vi "simple_acquisition.vi"() -> ()   [LabVIEW 2015]
uses:
  <vilib>/userdefined/High Color/IMAQdx.ctl
  <vilib>/vision/driver/NI_Vision_Acquisition_Software.lvlib
  <resource>/objmgr/imaqdx.rc
panel:
  in  "ExposureTimeRawValue":dbl(slide)=2237.4518320560815 scale=1.0..100000.0
  in  "File Path Control":path
  in  "Camera":T1="cam4"
  out "Image source":T2(plugin-control)
  in  "Acquire Image":bool
  in  "Image Name":string
  in  "Image Format":string(combo)=".png"
  in  "Stop Button":bool
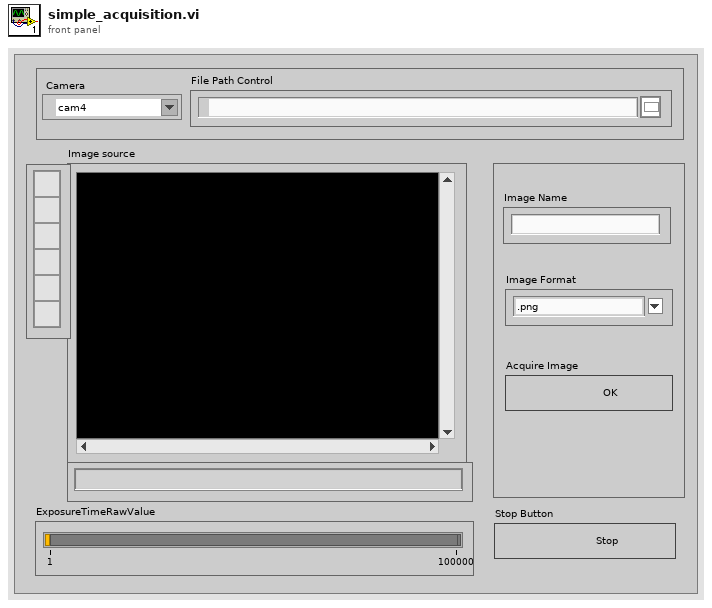
[diagram p1: front panel]
types:
  T1 = typedef "IMAQdx.ctl" = refnum<k21>
  T2 = typedef "IMAQ Image.ctl" = refnum<image>
  T3 = typedef "Image Type" = u32
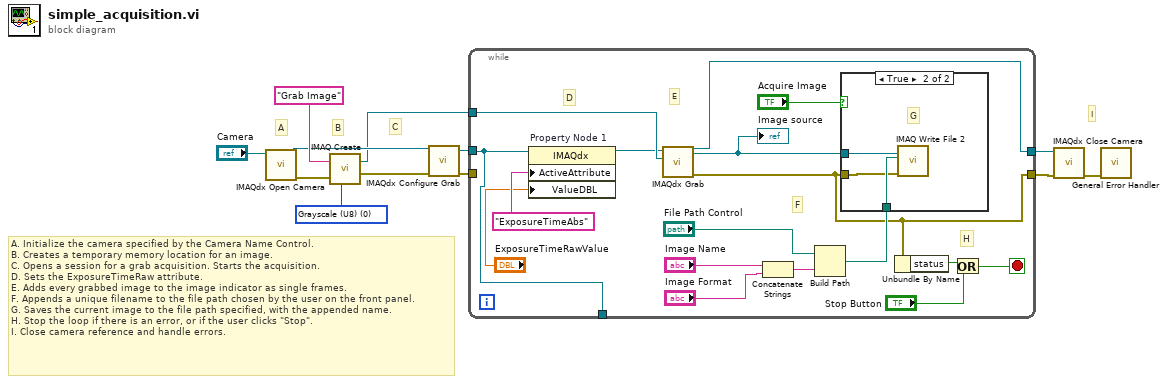
[diagram p0: block diagram]
diagram:
  w11 = T3 0 items=["Grayscale (U8)", "Grayscale (I16)", "Grayscale (SGL)", "Complex (CSG)", "RGB (U32)", "HSL (U32)", "RGB (U64)"] ("Image Type")
  # "I"
  # "C"
  # "A. Initialize the camera specified by the Camera Name Control.\nB. Creates a temporary memory location for an image.\nC. Opens a session for a grab acquisition. Starts the acquisition.\nD. Sets the ExposureTimeRaw attribute. \nE. Adds every grabbed image to the image indicator as single frames.\nF. Appends a unique filename to the file path chosen by the user on the front panel.\nG. Saves the current image to the file path specified, with the appended name.\nH. Stop the loop if there is an error, or if the user clicks \"Stop\".\nI. Close camera reference and handle errors."
  # "B"
  # "A"
  n1 = call <vilib>:"IMAQdx Open Camera.vi"("Session In"="Camera") -> ("error out"=w3:errorcluster, "Session Out"=w8:T1)  [unwired: 2 in, 7 out]
  n2 = call "IMAQ Create"("Image Name"="Grab Image", "Image Type"=w11, "error in (no error)"=w3) -> ("New Image"=w1:T2, "error out"=w10:errorcluster)  [unwired: 1 in, 1 out]
  n3 = call <vilib>:"IMAQdx Configure Grab.vi"("error in"=w10, "Session In"=w8) -> ("error out"=w2:errorcluster, "Session Out"=w4:T1)  [unwired: 8 out]
  n4 = while {
    tunnel: w2 -> [_]
    tunnel: w4 -> [w13]
    tunnel: [w19] -> w6
    tunnel: [w21] -> w5
    tunnel: w1 -> [w18]
    tunnel: [w13] -> _
    stop <- w23 stop-if-true
    # "H"
    # "F"
    # "E"
    # "D"
    n5 = property on="Property Node 1" class="IMAQdx"(reference=w13, "ActiveAttribute"="ExposureTimeAbs" ("String"), "ValueDBL"="ExposureTimeRawValue") -> (reference out=w17:T1)  [unwired: 1 in, 1 out]
    n6 = call <vilib>:"IMAQdx Grab.vi"("Image In"=w18, "Session In"=w17) -> ("error out"=w19:errorcluster, "Image Out"=w14:T2, "Session Out"=w21:T1)  [unwired: 2 in, 5 out]
    "Image source" <- w14
    n7 = Concatenate Strings("Image Name", "Image Format") -> (w29:string)
    n8 = Build Path(base path="File Path Control", name or relative path=w29) -> (appended path=w25:path)
    n9 = case shown="True" "Acquire Image" {
      tunnel: w14 -> [_ w30]
      tunnel: w25 -> [_ w32]
      tunnel: w19 -> [_ w31]
      frame False {
      }
      frame True {
        # "G"
        n10 = call-poly "IMAQ Write File 2"("error in (no error)"=w31, "File Path"=w32, "Image"=w30) -> ()  [unwired: 7 in, 2 out]
      }
    }
    n11 = Unbundle By Name(w19) -> ("status"=w24:bool)
    n12 = Or(x=w24, y="Stop Button") -> (x .or. y?=w23:bool)
  }
  n13 = call <vilib>:"IMAQdx Close Camera.vi"("error in"=w6, "Session In"=w5) -> ("error out"=w7:errorcluster)  [unwired: 9 out]
  n14 = call <vilib>:"General Error Handler.vi"("error in (no error)"=w7) -> ()  [unwired: 2 in, 13 out]
